vi "Set Test Signal Configuration.vi"(9 "signal configuration":refnum<class "SV Signal.lvclass">, 11 "variant in":variant) -> (3 "variant out":variant)   [LabVIEW 2017]
uses:
  <vilib>/addons/_NISVFA/_Generation/Signal Generation/SV Signal/SV Signal.lvclass
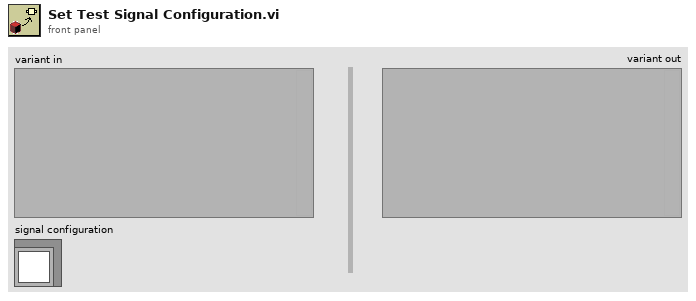
[diagram p1: front panel]
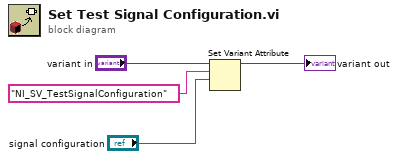
[diagram p0: block diagram]
diagram:
  n1 = Set Variant Attribute(Variant="variant in", name="NI_SV_TestSignalConfiguration", value="signal configuration") -> (Variant out=→"variant out":variant)  [unwired: 1 in, 2 out]
